vi "gui_T1_analysis -2017.07.24.vi"(6 "fitted_signal":T2, 8 "fit_parameters":T3, 9 "T1 curve":cluster{dbl[], "dark_time_us":dbl[]}, 10 "T1_parameters":T1, 11 "timetags":u32[][](array[numeric])) -> ()   [LabVIEW 2014]
panel:
  out "sampling_mode":enum16{"Normal", "Sweep"}(ring)
  out "quality":bool
  out "mse":dbl caption="Mean Square Error" format="%#.4g"
  out "T1_us":dbl format="%#.3g"
  out "T1 curves":cluster{dbl[], "dark_time_us":dbl[]}[](graph)
  in  "correction_us":dbl caption="Delay"
  out "stop_count_photon":u32(colorbox)=16776704 caption="Stop Count & photon"
  out "stop_count":u32(colorbox)=6618880 caption="Stop Count"
  out "start_count_photon":u32(colorbox)=14417925 caption="Start Count & photon"
  out "start_count":u32(colorbox)=255 caption="Start Count"
  out "photon":u32(colorbox)=16448250 caption="Photon"
  out "noPhoton":u32(colorbox) caption="No Photon"
  out "photons_chart":u32[][](graph)
  in  "load_file":bool
  in  "refit":bool
  in  "read_width_us":dbl=0.3 caption="Width" min=0.0 max=10000.0 format="%#.3f"
  out "read_delay_us":dbl caption="Delay"
  out "min_step":dbl format="%#.3f"
  out "q_samples":i32=100
  out "dt_stop_us":dbl=1.0
  out "dt_start_us":dbl=0.1
  in  "stop":bool
  out "repetitions":i32=100 caption="Repetitions" min=1 step=1
  out "pulse_width_us":dbl=3.0 caption="Pulse width"
  # "Dark time [us]"
  # "*"
  # "*"
  # "us"
  # "*read_width_us and correction_us have to be multiple of 10ns\n*** start and stop markers are inside the detection gate. [start, stop]"
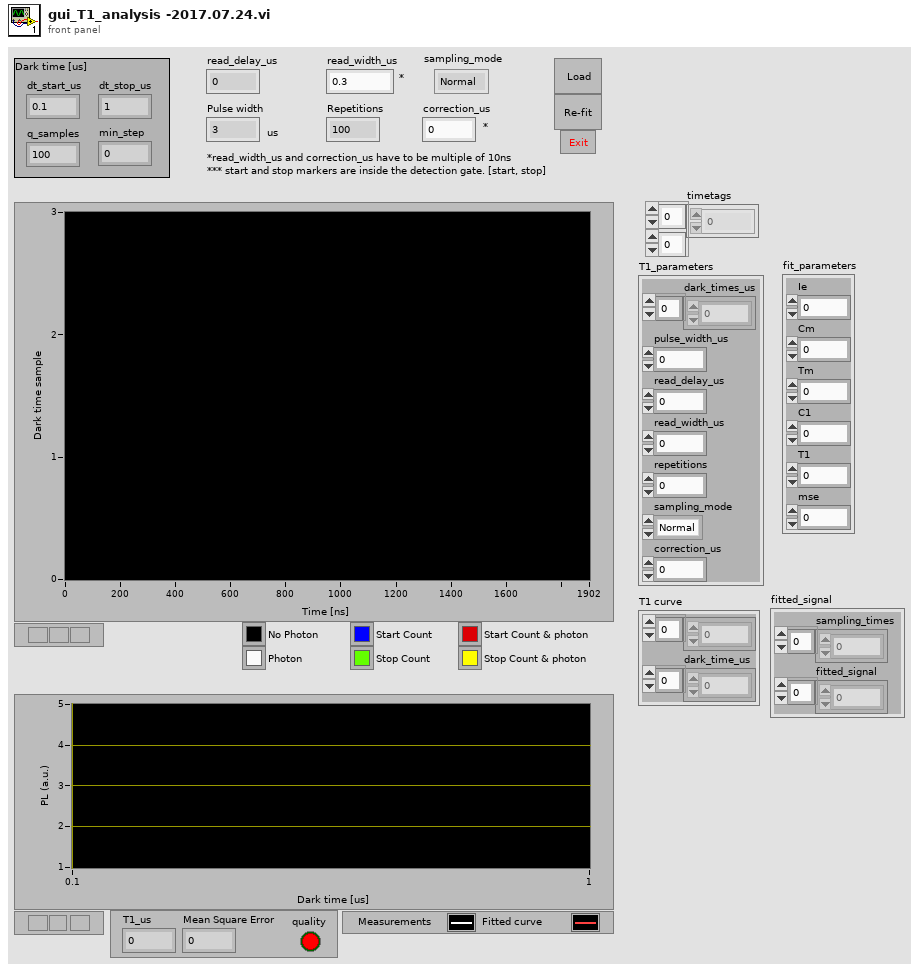
[diagram p1: front panel]
types:
  T1 = cluster{"dark_times_us":dbl[], "pulse_width_us":dbl, "read_delay_us":dbl, "read_width_us":dbl, "repetitions":i32, "sampling_mode":enum16{"Normal", "Sweep"}, "correction_us":dbl}
  T2 = cluster{"sampling_times":dbl[], "fitted_signal":dbl[]}
  T3 = cluster{"Ie":dbl, "Cm":dbl, "Tm":dbl, "C1":dbl, "T1":dbl, "mse":dbl}
  T4 = enum16{"standby", "doT1", "abort", "save", "re-fit", "load"}
  T5 = enum16{"standby", "doT1", "abort", "save", "re-fit", "load", "refresh"}
  T6 = cluster{"sampling_times":dbl[], "fitted_signal":dbl[]}[]
  T7 = cluster{"dark_times":dbl[], "fitted_signal":dbl[]}
  T8 = cluster{"dark_times_us":dbl[], "measured_signal":dbl[]}
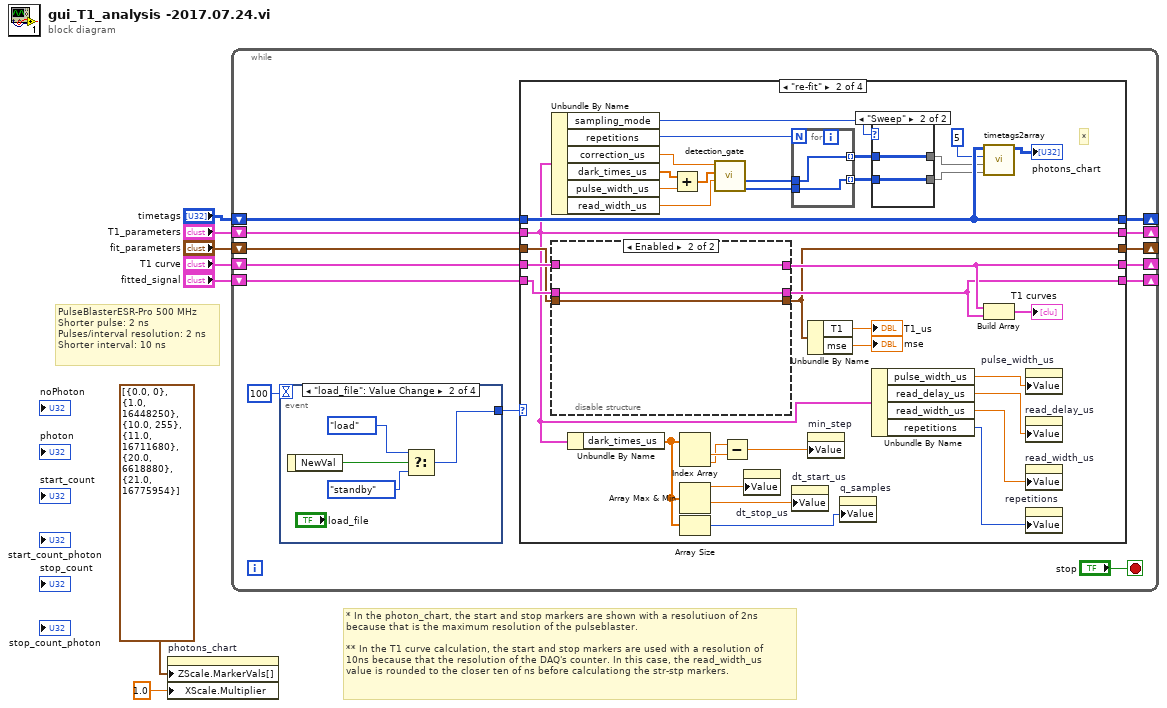
[diagram p0: block diagram]
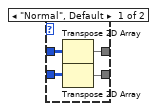
[diagram p3: hidden frame]
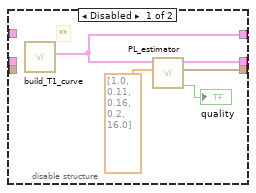
[diagram p4: hidden frame]
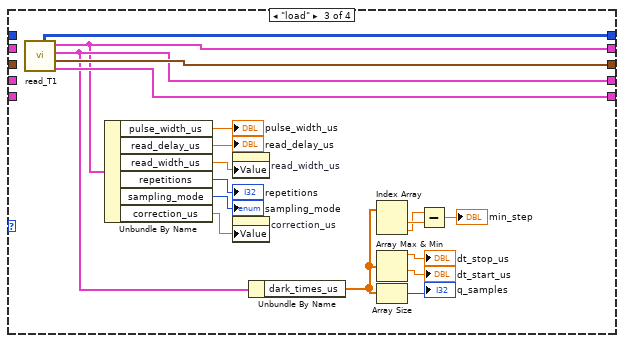
[diagram p5: hidden frame]
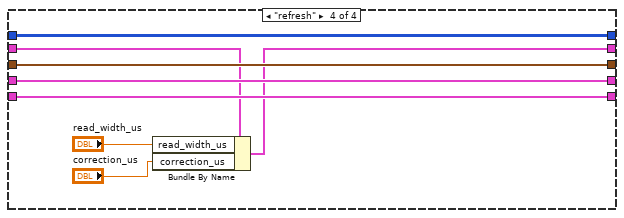
[diagram p6: hidden frame]
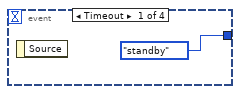
[diagram p7: hidden frame]
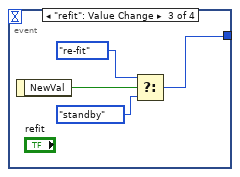
[diagram p8: hidden frame]
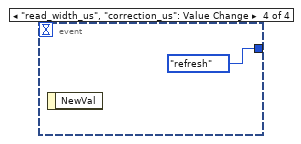
[diagram p9: hidden frame]
diagram:
  # "* In the photon_chart, the start and stop markers are shown with a resolutiuon of 2ns \nbecause that is the maximum resolution of the pulseblaster.\n\n** In the T1 curve calculation, the start and stop markers are used with a resolution of\n10ns because that the resolution of the DAQ's counter. In this case, the read_width_us\nvalue is rounded to the closer ten of ns before calculationg the str-stp markers."
  # "PulseBlasterESR-Pro 500 MHz \nShorter pulse: 2 ns\nPulses/interval resolution: 2 ns\nShorter interval: 10 ns"
  n1 = property on="photons_chart" class="IntGraph (strict)"("ZScale.MarkerVals[]"=cluster{dbl, u32}[] [{0.0, 0}, {1.0, 16448250}, {10.0, 255}, {11.0, 16711680}, {20.0, 6618880}, {21.0, 16775954}] ("Z Scale.Marker Values[]"), "XScale.Multiplier"=1.0 ("X Scale.Offset and Multiplier:Multiplier")) -> ()  [unwired: 2 in, 2 out]
  n2 = while {
    shift-right: [w10] -> _
    shift-left: "T1_parameters" -> [w17]
    shift-right: [w9] -> _
    shift-left: "fit_parameters" -> [w16]
    shift-right: [w8] -> _
    shift-left: "T1 curve" -> [w15]
    shift-right: [w14] -> _
    shift-left: "fitted_signal" -> [w13]
    shift-right: [w11] -> _
    shift-left: "timetags" -> [w12]
    stop <- "stop" stop-if-true
    n3 = event shown="[1] \"load_file\": Value Change" {
      selector: _ -> [_ _ _ _]
      dyn-events: _ -> [_ _ _ _]
      timeout: 100 -> [_ _ _ _]
      tunnel: [T4."standby" w107 w112 T5."refresh"] -> w18
      event Timeout {
        n4 = event-data() -> ()  [unwired: 1 in, 1 out]
      }
      event "load_file": Value Change {
        n5 = event-data() -> ("NewVal"=w108:bool)  [unwired: 1 in]
        n6 = Select(t=T4."load", s=w108, f=T4."standby") -> (s? t:f=w107:T4)
      }
      event "refit": Value Change {
        n7 = event-data() -> ("NewVal"=w113:bool)  [unwired: 1 in]
        n8 = Select(t=T4."re-fit", s=w113, f=T4."standby") -> (s? t:f=w112:T4)
      }
      event "read_width_us", "correction_us": Value Change {
        n9 = event-data() -> ()  [unwired: 1 in, 1 out]
      }
    }
    n10 = case shown="\"re-fit\"" w18 {
      tunnel: w17 -> [w25 w39 _ w100]
      tunnel: w16 -> [w24 w51 _ w103]
      tunnel: w15 -> [w23 w53 _ w102]
      tunnel: [w22 w59 w96 w101] -> w14
      tunnel: w13 -> [w22 w52 _ w101]
      tunnel: [w21 w55 w79 w104] -> w11
      tunnel: w12 -> [w21 w55 _ w104]
      tunnel: [w25 w39 w82 w99] -> w10
      tunnel: [w24 w58 w95 w103] -> w9
      tunnel: [w23 w60 w91 w102] -> w8
      frame "standby", Default {
      }
      frame "re-fit" {
        # "*"
        n11 = Unbundle By Name(w39) -> ("sampling_mode"=w28:enum16{"Normal", "Sweep"}, "repetitions"=w32:i32, "correction_us"=w34:dbl, "dark_times_us"=w33:dbl[], "pulse_width_us"=w37:dbl, "read_width_us"=w38:dbl)
        n12 = disable-structure shown="Enabled" {
          disable-tunnel: [w75 w78] -> w60
          disable-tunnel: [w74 w77] -> w59
          disable-tunnel: [w73 w76] -> w58
          disable-tunnel: w53 -> [_ w78]
          disable-tunnel: w52 -> [_ w77]
          disable-tunnel: w51 -> [_ w76]
          frame Disabled {
            # "**"
            n13 = call "build_T1_curve.vi"() -> ("T1 curve"=w75:cluster{dbl[], "dark_time_us":dbl[]})  [unwired: 8 in, 3 out]
            n14 = call "PL_estimator.vi"("initial parameters"=dbl[] [1.0, 0.11, 0.16, 0.2, 16.0], "measured_signal"=w75) -> ("quality_check"=→"quality":bool, "fit_parameters"=w73:T3, "fitted_signal"=w74:T2)  [unwired: 7 in]
          }
          frame Enabled {
          }
        }
        n15 = Unbundle By Name(w39) -> ("dark_times_us"=w48:dbl[])
        n16 = Add(x=w33, y=w37) -> (x+y=w31:dbl[])
        n17 = Index Array(array=w48) -> (element #1=w50:dbl, element #2=w49:dbl)  [unwired: 2 in]
        n18 = Array Max & Min(array=w48) -> (max value=w47:dbl, min value=w46:dbl)  [unwired: 2 out]
        n19 = Array Size(array=w48) -> (size(s)=w45:i32)
        n20 = call "detection_gate.vi"("read_width_us"=w38, "pulse_period_us"=w31, "correction_us"=w34) -> ("start_read"=w35:u32[], "stop_read"=w36:u32[])  [unwired: 7 in]
        n21 = Subtract(x=w49, y=w50) -> (x-y=w44:dbl)
        n22 = property on="dt_stop_us" class="DigNum (strict)"("Value"=w47) -> ()  [unwired: 2 in, 2 out]
        n23 = for {
          N: w32 -> [_]
          tunnel: w36 -> [w70]
          tunnel: w35 -> [w69]
          tunnel: [w70] -> w29 mode=indexing
          tunnel: [w69] -> w30 mode=indexing
        }
        n24 = property on="dt_start_us" class="DigNum (strict)"("Value"=w46) -> ()  [unwired: 2 in, 2 out]
        n25 = Unbundle By Name(w58) -> ("T1"=→"T1_us":dbl, "mse"=→"mse":dbl)
        n26 = property on="min_step" class="DigNum (strict)"("Value"=w44) -> ()  [unwired: 2 in, 2 out]
        n27 = property on="q_samples" class="DigNum (strict)"("Value"=w45) -> ()  [unwired: 2 in, 2 out]
        n28 = case shown="\"Sweep\"" w28 {
          tunnel: w30 -> [w66 w67]
          tunnel: w29 -> [w63 w68]
          tunnel: [w64 w68] -> w26
          tunnel: [w65 w67] -> w27
          frame "Normal", Default {
            n29 = Transpose 2D Array(2D array=w63) -> (transposed array=w64:u32[][])
            n30 = Transpose 2D Array(2D array=w66) -> (transposed array=w65:u32[][])
          }
          frame "Sweep" {
          }
        }
        n31 = Unbundle By Name(w39) -> ("pulse_width_us"=w43:dbl, "read_delay_us"=w42:dbl, "read_width_us"=w41:dbl, "repetitions"=w40:i32)
        n32 = call "timetags2array.vi"("start_read"=w27, "stop_read"=w26, "pixels per count"=u32 5, "timetags"=w55) -> ("photons_chart"=→"photons_chart":u32[][])  [unwired: 7 in]
        n33 = Build Array(w60, w59) -> (→"T1 curves":T6)
        n34 = property on="pulse_width_us" class="DigNum (strict)"("Value"=w43) -> ()  [unwired: 2 in, 2 out]
        n35 = property on="read_delay_us" class="DigNum (strict)"("Value"=w42) -> ()  [unwired: 2 in, 2 out]
        n36 = property on="read_width_us" class="DigNum (strict)"("Value"=w41) -> ()  [unwired: 2 in, 2 out]
        n37 = property on="repetitions" class="DigNum (strict)"("Value"=w40) -> ()  [unwired: 2 in, 2 out]
      }
      frame "load" {
        n38 = call "read_T1.vi"() -> ("fitted_signal"=w96:T7, "fit_parameters"=w95:T3, "T1_curve"=w91:T8, "T1_parameters"=w82:T1, "timetags"=w79:u32[][])  [unwired: 7 in]
        n39 = Unbundle By Name(w82) -> ("pulse_width_us"=→"pulse_width_us":dbl, "read_delay_us"=→"read_delay_us":dbl, "read_width_us"=w83:dbl, "repetitions"=→"repetitions":i32, "sampling_mode"=→"sampling_mode":enum16{"Normal", "Sweep"}, "correction_us"=w80:dbl)
        n40 = property on="read_width_us" class="DigNum (strict)"("Value"=w83) -> ()  [unwired: 2 in, 2 out]
        n41 = property on="correction_us" class="DigNum (strict)"("Value"=w80) -> ()  [unwired: 2 in, 2 out]
        n42 = Unbundle By Name(w91) -> ("dark_times_us"=w87:dbl[])
        n43 = Index Array(array=w87) -> (element #1=w86:dbl, element #2=w85:dbl)  [unwired: 2 in]
        n44 = Array Max & Min(array=w87) -> (max value=→"dt_stop_us":dbl, min value=→"dt_start_us":dbl)  [unwired: 2 out]
        n45 = Array Size(array=w87) -> (size(s)=→"q_samples":i32)
        n46 = Subtract(x=w85, y=w86) -> (x-y=→"min_step":dbl)
      }
      frame "refresh" {
        n47 = Bundle By Name(cluster=w100, "read_width_us"="read_width_us", "correction_us"="correction_us") -> (w99:T1)
      }
    }
  }
